vi "variant2data_b.vi"() -> (7 "number of dimensions":i32, 8 "Size":u32, 10 "Variant Data Type":T2)   [LabVIEW 2019]
doc: "This example uses some of the Variant utility VIs to determine the datatype contained in a variant"
uses:
  <vilib>/Utility/VariantDataType/Type.ctl
  <vilib>/Utility/Data Type/Type Definitions/Data Type.ctl
  <vilib>/Utility/Data Type/NI_Data Type.lvlib
  <vilib>/Utility/VariantDataType/VariantType.lvlib
panel:
  out "Numeric":dbl
  out "data":T1
  out "ArrayElement":variant
  # "Overview:This example uses some of the Variant utility VIs to determine the datatype contained in a variant.\nRequirement: LabVIEW 2012 (or compatible)\nInstructions:\nRun the VI"
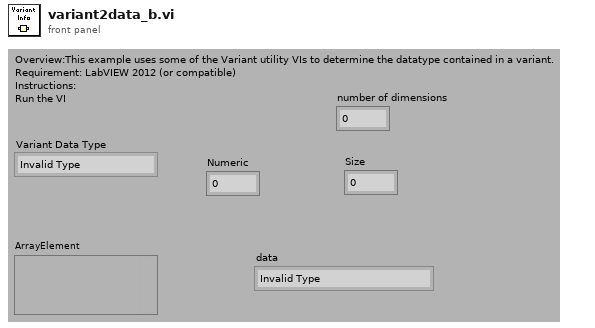
[diagram p1: front panel]
types:
  T1 = typedef "NI_Data Type.lvlib/Data Type.ctl" = enum8{"Invalid Type", "Void", "I8", "I16", "I32", "I64", "U8", "U16", "U32", "U64", "Single Float", "Double Float", "Extended Float", "Single Complex", "Double Complex", "Extended Complex", "Enum U8", "Enum U16", "Enum U32", "Enum U64", "Single Float With Unit", "Double Float With Unit", "Extended Float With Unit", "Single Complex with Unit", "Double Complex with Unit", "Extended Complex with Unit", "Boolean", "String", "Path", "Picture", "Tag", "Array", "Cluster", "Variant", "LV Variant", "Waveform", "Timestamp", "Digital Waveform", "Digital Data", "ExpressData", "Refnum", "External Data", "VI", "Poly VI", "LabVIEW Class Instance", "Fixed Point", "Set Collection", "Map Collection"}
  T2 = typedef "VariantType.lvlib/Type.ctl" = enum8{"Invalid Type", "Void", "I8", "I16", "I32", "I64", "U8", "U16", "U32", "U64", "Single Float", "Double Float", "Extended Float", "Single Complex", "Double Complex", "Extended Complex", "Enum U8", "Enum U16", "Enum U32", "Enum U64", "Single Float With Unit", "Double Float With Unit", "Extended Float With Unit", "Single Complex with Unit", "Double Complex with Unit", "Extended Complex with Unit", "Boolean", "String", "Path", "Picture", "Tag", "Array", "Cluster", "Variant", "LV Variant", "Waveform", "Timestamp", "Digital Waveform", "Digital Data", "ExpressData", "Refnum", "External Data", "VI", "Poly VI", "LabVIEW Class Instance", "Fixed Point"}
  T3 = typedef "NI_Data Type.lvlib/Memory Info.ctl" = cluster{"Type":T4, "Size":u32}
  T4 = typedef "NI_Data Type.lvlib/Memory Type.ctl" = enum16{"Variable", "Fixed", "Bounded"}
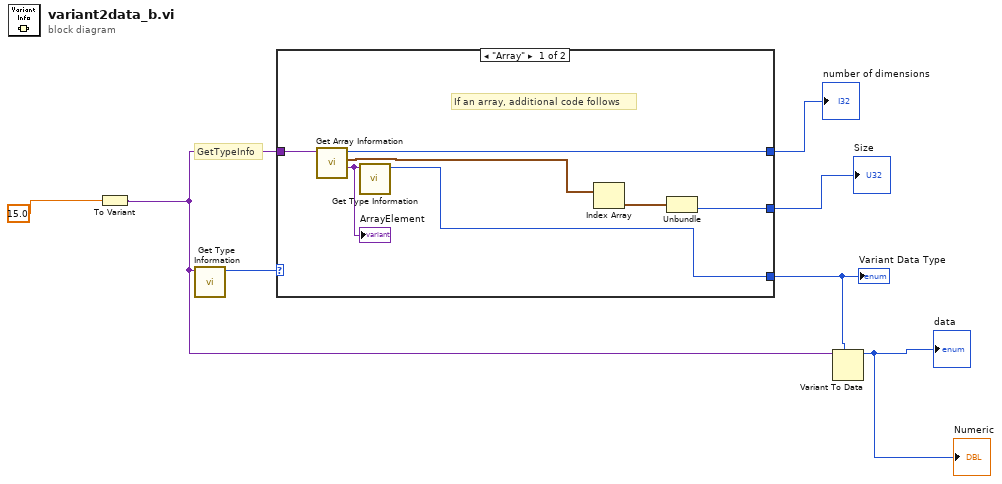
[diagram p0: block diagram]
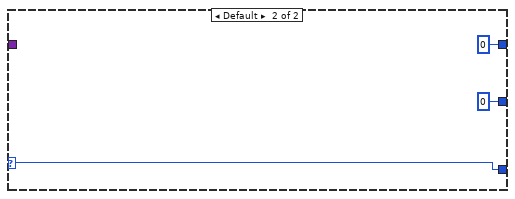
[diagram p2: hidden frame]
diagram:
  # "GetTypeInfo"
  n1 = To Variant(anything=15.0) -> (Variant=w3:variant)
  n2 = call <vilib>:"Get Type Information.vi"("variant"=w3) -> ("type"=w7:T1)  [unwired: 6 in, 4 out]
  n3 = case shown="\"Array\"" w7 {
    selector: w7 -> [_ w15]
    tunnel: w3 -> [w14 _]
    tunnel: [w8 w15] -> w4
    tunnel: [w12 0 ("number of dimensions")] -> w6
    tunnel: [w9 u32 0 ("Size")] -> w5
    frame "Array" {
      # "If an array, additional code follows"
      n4 = call <vilib>:"Get Array Information.vi"("variant"=w14) -> ("array element data type"=w13:variant, "array lengths"=w11:T3[], "number of dimensions"=w12:i32)  [unwired: 7 in, 1 out]
      "ArrayElement" <- w13
      n5 = call <vilib>:"Get Type Information.vi"("variant"=w13) -> ("type"=w8:T1)  [unwired: 6 in, 4 out]
      n6 = Index Array(array=w11) -> (element=w10:T3)  [unwired: 1 in]
      n7 = Unbundle(w10) -> ("Size"=w9:u32)  [unwired: 1 out]
    }
    frame Default {
    }
  }
  "Variant Data Type" <- w4
  "number of dimensions" <- w6
  "Size" <- w5
  n8 = Variant To Data(type=w4, Variant=w3) -> (data=→"data" →"Numeric":T1)  [unwired: 1 in, 1 out]
